vi "1D Array to StrPath.vi"(1 "File Path String Array":string[](array[string]), 2 "Delimiter":string) -> (0 "Path string":string)   [LabVIEW 2019, in "TLCD Test Class.lvclass"]
uses:
  TLCD Test Class.lvclass
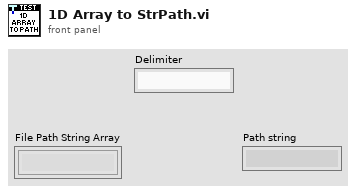
[diagram p1: front panel]
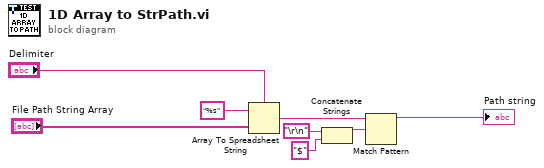
[diagram p0: block diagram]
diagram:
  n1 = Array To Spreadsheet String(delimiter (Tab)="Delimiter", array="File Path String Array", 3:"%s" ("format string")) -> (spreadsheet string=w8:string)
  n2 = Concatenate Strings("\r\n", "$" ("Substring")) -> (w7:string)
  n3 = Match Pattern(string=w8, regular expression=w7) -> (before substring=→"Path string":string)  [unwired: 1 in, 3 out]
